vi "Timing_test_code.vi"() -> ()   [LabVIEW 2017]
uses:
  <vilib>/DAQmx/write.llb/DAQmx Write (Digital 1D Wfm NChan NSamp).vi
  <vilib>/DAQmx/read.llb/DAQmx Read (Analog 1D Wfm NChan NSamp).vi
  <vilib>/DAQmx/create/channels.llb/DAQmx Create Channel (DO-Digital Output).vi
  <vilib>/DAQmx/configure/timing.llb/DAQmx Timing (Sample Clock).vi
  <vilib>/DAQmx/create/channels.llb/DAQmx Create Channel (AI-Current-Basic).vi
  <vilib>/DAQmx/create/channels.llb/DAQmx Create Channel (AI-Voltage-Basic).vi
  <vilib>/DAQmx/create/channels.llb/DAQmx Create Channel (AI-Temperature-Thermocouple).vi
  <vilib>/Waveform/DWDTOps.llb/DWDT Uncompress Digital.vi
  <vilib>/DAQmx/miscellaneous.llb/DAQmx Fill In Error Info.vi
  <resource>/objmgr/daqmx.rc
panel:
  out "Waveform Graph":waveform(dbl)[](graph)
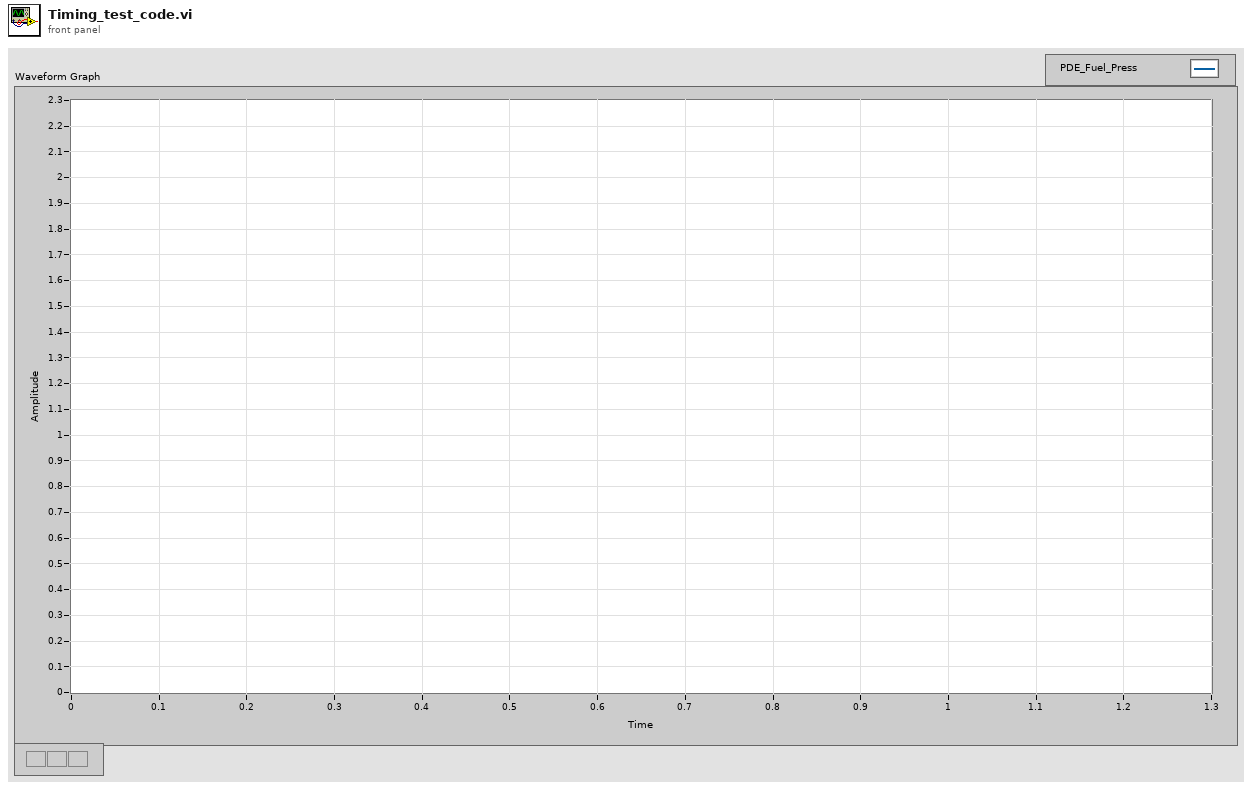
[diagram p1: front panel]
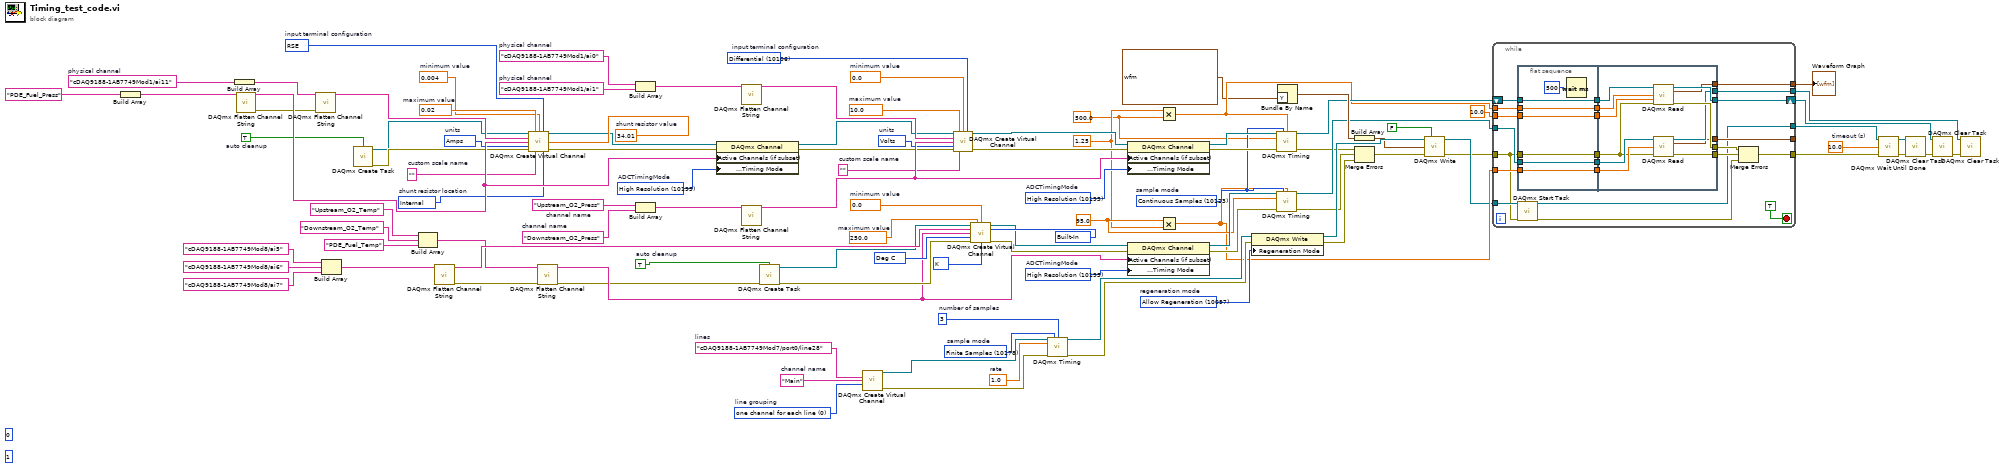
[diagram p0: block diagram]
diagram:
  (unwired) u32 1 ("number of ticks")
  (unwired) u8 0 ("trigger ID")
  w14 = 500.0 ("rate")
  w75 = 10195 items=["High Resolution"=10195, "High Speed"=14712, "Best 50 Hz Rejection"=14713, "Best 60 Hz Rejection"=14714]  # ADCTimingMode
  w87 = "Downstream_O2_Press"  # channel name
  w84 = "cDAQ9188-1AB7749Mod1/ai1"  # physical channel
  w74 = 10106 items=["default"=-1, "RSE"=10083, "NRSE"=10078, "Differential"=10106, "Pseudodifferential"=12529]  # input terminal configuration
  w89 = 10348 items=["Volts"=10348, "From Custom Scale"=10065]  # units
  w88 = "Upstream_O2_Press"  # channel name
  w73 = ""  # custom scale name
  w72 = 0.0  # minimum value
  w71 = 10.0  # maximum value
  w83 = "cDAQ9188-1AB7749Mod1/ai0"  # physical channel
  w69 = "cDAQ9188-1AB7749Mod1/ai11"  # physical channel
  w76 = 10123 items=["Finite Samples"=10178, "Continuous Samples"=10123, "Hardware Timed Single Point"=12522]  # sample mode
  w49 = 10195 items=["High Resolution"=10195, "High Speed"=14712, "Best 50 Hz Rejection"=14713, "Best 60 Hz Rejection"=14714]  # ADCTimingMode
  w50 = 10083 items=["default"=-1, "RSE"=10083, "NRSE"=10078, "Differential"=10106, "Pseudodifferential"=12529]  # input terminal configuration
  w51 = 10342 items=["Amps"=10342, "From Custom Scale"=10065]  # units
  w52 = 34.01  # shunt resistor value
  w53 = 10200 items=["Internal"=10200, "External"=10167]  # shunt resistor location
  w55 = ""  # custom scale name
  w56 = 0.004  # minimum value
  w57 = 0.02  # maximum value
  w59 = TRUE  # auto cleanup
  w46 = 10143 items=["Deg C"=10143, "Deg F"=10144, "Kelvins"=10325, "Deg R"=10145, "From Custom Scale"=10065] ("units")
  w45 = 10073 items=["J"=10072, "K"=10073, "N"=10077, "R"=10082, "S"=10085, "T"=10086, "B"=10047, "E"=10055] ("thermocouple type")
  w44 = 10200 items=["Built-In"=10200, "Constant Value"=10116, "Channel"=10113] ("cjc source")
  w35 = 10195 items=["High Resolution"=10195, "High Speed"=14712, "Best 50 Hz Rejection"=14713, "Best 60 Hz Rejection"=14714]  # ADCTimingMode
  w38 = 0.0  # minimum value
  w39 = 250.0  # maximum value
  w41 = TRUE  # auto cleanup
  w21 = 1.25 ("Sampling Time")
  w22 = 95.0 ("Temperature Freq")
  w98 = 0 items=["one channel for each line", "one channel for all lines"]  # line grouping
  w97 = "Main"  # channel name
  w99 = "cDAQ9188-1AB7749Mod7/port0/line28"  # lines
  w104 = 10097 items=["Allow Regeneration"=10097, "Do Not Allow Regeneration"=10158]  # regeneration mode
  w94 = 10178 items=["Finite Samples"=10178, "Continuous Samples"=10123, "Hardware Timed Single Point"=12522]  # sample mode
  w95 = 3  # number of samples
  w93 = 1.0  # rate
  w100 = 10.0  # timeout (s)
  n1 = Build Array("PDE_Fuel_Press" ("element")) -> (w62:string[])
  n2 = Build Array(w69) -> (w64:string[])
  n3 = call <vilib>:"DAQmx Flatten Channel String.vi"("names in"=w62) -> ("names out"=w63:string, "error out"=w24:errorcluster)  [unwired: 13 in]
  n4 = call <vilib>:"DAQmx Flatten Channel String.vi"("names in"=w64, "error in"=w24) -> ("names out"=w61:string)  [unwired: 12 in, 1 out]
  n5 = Build Array("cDAQ9188-1AB7749Mod8/ai5" ("element"), "cDAQ9188-1AB7749Mod8/ai6" ("element"), "cDAQ9188-1AB7749Mod8/ai7" ("element")) -> (w47:string[])
  n6 = call <vilib>:"DAQmx Create Task.vi"("auto cleanup"=w59) -> ("task out"=w58:refnum<k21>, "error out"=w60:errorcluster)  [unwired: 4 in, 9 out]
  n7 = Build Array("Upstream_O2_Temp" ("name to assign"), "Downstream_O2_Temp" ("name to assign"), "PDE_Fuel_Temp" ("name to assign")) -> (w31:string[])
  n8 = call <vilib>:"DAQmx Flatten Channel String.vi"("names in"=w47) -> ("names out"=w43:string, "error out"=w23:errorcluster)  [unwired: 13 in]
  n9 = call-poly <vilib>:"DAQmx Create Virtual Channel.vi"("task in"=w58, "maximum value"=w57, "minimum value"=w56, "input terminal configuration"=w50, "physical channels"=w61, "name to assign"=w63, "external shunt resistor value"=w52, "units"=w51, "error in"=w60, "custom scale name"=w55, "shunt resistor location"=w53) -> ("task out"=w48:refnum<k21>, "error out"=w54:errorcluster)  [unwired: 3 out]
  n10 = call <vilib>:"DAQmx Flatten Channel String.vi"("names in"=w31, "error in"=w23) -> ("names out"=w27:string, "error out"=w26:errorcluster)  [unwired: 12 in]
  n11 = Build Array(w83, w84) -> (w82:string[])
  n12 = Build Array(w88, w87) -> (w86:string[])
  n13 = property class="DAQmx Channel"(reference=w48, error in=w54, "Active Channels (if subset)"=w63, "Analog Input:General Properties:Digitizer/ADC:Timing Mode"=w49) -> (reference out=w78:refnum<k21>, error out=w79:errorcluster)
  n14 = call <vilib>:"DAQmx Flatten Channel String.vi"("names in"=w82) -> ("names out"=w85:string)  [unwired: 13 in, 1 out]
  n15 = call <vilib>:"DAQmx Flatten Channel String.vi"("names in"=w86) -> ("names out"=w92:string)  [unwired: 13 in, 1 out]
  n16 = call <vilib>:"DAQmx Create Task.vi"("auto cleanup"=w41, "error in"=w26) -> ("task out"=w40:refnum<k21>, "error out"=w42:errorcluster)  [unwired: 3 in, 9 out]
  n17 = call-poly <vilib>:"DAQmx Create Virtual Channel.vi"("lines"=w99, "name to assign"=w97, "line grouping"=w98) -> ("task out"=w12:refnum<k21>, "error out"=w13:errorcluster)  [unwired: 11 in]
  n18 = call-poly <vilib>:"DAQmx Create Virtual Channel.vi"("task in"=w78, "maximum value"=w71, "minimum value"=w72, "input terminal configuration"=w74, "physical channels"=w85, "name to assign"=w92, "units"=w89, "error in"=w79, "custom scale name"=w73) -> ("task out"=w90:refnum<k21>, "error out"=w91:errorcluster)  [unwired: 5 in]
  n19 = call-poly <vilib>:"DAQmx Create Virtual Channel.vi"("task in"=w40, "maximum value"=w39, "minimum value"=w38, "physical channels"=w43, "cjc source"=w44, "name to assign"=w27, "units"=w46, "error in"=w42, "thermocouple type"=w45) -> ("task out"=w34:refnum<k21>, "error out"=w37:errorcluster)  [unwired: 5 in]
  n20 = call-poly <vilib>:"DAQmx Timing.vi"("task/channels in"=w12, "sample mode"=w94, "samples per channel"=w95, "rate"=w93, "error in"=w13) -> ("task out"=w105:refnum<k21>, "error out"=w106:errorcluster)  [unwired: 9 in]
  n21 = property class="DAQmx Channel"(reference=w90, error in=w91, "Active Channels (if subset)"=w92, "Analog Input:General Properties:Digitizer/ADC:Timing Mode"=w75) -> (reference out=w77:refnum<k21>, error out=w80:errorcluster)
  n22 = property class="DAQmx Channel"(reference=w34, error in=w37, "Active Channels (if subset)"=w27, "Analog Input:General Properties:Digitizer/ADC:Timing Mode"=w35) -> (reference out=w33:refnum<k21>, error out=w36:errorcluster)
  n23 = Multiply(x=w21, y=w14) -> (x*y=w25:dbl)
  n24 = Multiply(x=w22, y=w21) -> (x*y=w18:dbl)
  n25 = property class="DAQmx Write"(reference=w105, error in=w106, "Regeneration Mode"=w104) -> (reference out=w103:refnum<k21>, error out=w15:errorcluster)
  n26 = call-poly <vilib>:"DAQmx Timing.vi"("task/channels in"=w77, "sample mode"=w76, "samples per channel"=w25, "rate"=w14, "error in"=w80) -> ("task out"=w65:refnum<k21>, "error out"=w17:errorcluster)  [unwired: 2 in, 7 out]
  n27 = call-poly <vilib>:"DAQmx Timing.vi"("task/channels in"=w33, "sample mode"=w76, "samples per channel"=w18, "rate"=w22, "error in"=w36) -> ("task out"=w20:refnum<k21>, "error out"=w16:errorcluster)  [unwired: 2 in, 7 out]
  n28 = Bundle By Name("Y"=digitaldata {"transitions"=[], "data"=[[0], [1], [0], [0]]}) -> (w96:digitalwaveform)  [unwired: 1 in]
  n29 = Build Array(w96) -> (w102:digitalwaveform[])
  n30 = Merge Errors(w17, w16, w15) -> (w2:errorcluster)
  n31 = call-poly <vilib>:"DAQmx Write.vi"("task/channels in"=w103, "auto start"=FALSE, "data"=w102, "error in"=w2) -> ("task out"=w4:refnum<k21>, "error out"=w3:errorcluster)  [unwired: 9 in, 1 out]
  n32 = while {
    tunnel: 10.0 ("timeout") -> [w129]
    tunnel: w25 -> [w126]
    shift-right: [w128] -> w32
    shift-left: w65 -> [w127]
    tunnel: w20 -> [w125]
    tunnel: [w122] -> w19
    tunnel: w18 -> [w121]
    tunnel: [w120] -> _
    tunnel: [w119] -> w11
    tunnel: w4 -> [w117]
    tunnel: [w115] -> w7
    tunnel: w3 -> [w114]
    tunnel: [w113] -> w1
    stop <- TRUE stop-if-true
    n33 = flat-sequence {
      tunnel: w114 -> [w131]
      tunnel: w121 -> [w132]
      tunnel: w125 -> [w133]
      tunnel: w126 -> [w134]
      tunnel: w127 -> [w135]
      tunnel: w129 -> [w136]
      tunnel: [w136] -> w112
      tunnel: [w135] -> w111
      tunnel: [w134] -> w110
      tunnel: [w133] -> w109
      tunnel: [w132] -> w108
      tunnel: [w131] -> w107
      tunnel: [w147] -> w128
      tunnel: [w143] -> w124
      tunnel: [w142] -> w123
      tunnel: [w141] -> w122
      tunnel: [w139] -> w120
      tunnel: [w138] -> w119
      tunnel: w112 -> [w148]
      tunnel: w111 -> [w146]
      tunnel: w110 -> [w145]
      tunnel: w109 -> [w144]
      tunnel: w108 -> [w140]
      tunnel: w107 -> [w137]
      frame #0 {
        n34 = Wait (ms)(milliseconds to wait=u32 500) -> ()  [unwired: 1 out]
      }
      frame #1 {
        n35 = call-poly <vilib>:"DAQmx Read.vi"("task/channels in"=w146, "number of samples per channel"=w145, "timeout"=w148, "error in"=w137) -> ("task out"=w147:refnum<k21>, "data"=w138:waveform(dbl)[], "error out"=w143:errorcluster)  [unwired: 9 out]
        n36 = call-poly <vilib>:"DAQmx Read.vi"("task/channels in"=w144, "number of samples per channel"=w140, "error in"=w137) -> ("task out"=w141:refnum<k21>, "data"=w139:waveform(dbl)[], "error out"=w142:errorcluster)  [unwired: 1 in, 9 out]
      }
    }
    n37 = call <vilib>:"DAQmx Start Task.vi"("task/channels in"=w117, "error in"=w114) -> ("task out"=w115:refnum<k21>, "error out"=w116:errorcluster)  [unwired: 12 in]
    n38 = Merge Errors(w124, w123, w116) -> (w113:errorcluster)
  }
  "Waveform Graph" <- w11
  n39 = call <vilib>:"DAQmx Wait Until Done.vi"("task/channels in"=w7, "timeout (sec)"=w100, "error in"=w1) -> ("task out"=w101:refnum<k21>, "error out"=w5:errorcluster)  [unwired: 11 in]
  n40 = call <vilib>:"DAQmx Clear Task.vi"("task in"=w101, "error in"=w5) -> ("error out"=w9:errorcluster)  [unwired: 13 in]
  n41 = call <vilib>:"DAQmx Clear Task.vi"("task in"=w32, "error in"=w9) -> ("error out"=w8:errorcluster)  [unwired: 13 out]
  n42 = call <vilib>:"DAQmx Clear Task.vi"("task in"=w19, "error in"=w8) -> ()  [unwired: 14 out]
